vi "Create StringMsg.vi"(8 "error in (no error)":errorcluster, 10 "Message Data":string, 11 "Message Name":string) -> (0 "error out":errorcluster, 3 "StringMsg out":refnum<class "StringMsg.lvclass">)   [LabVIEW 2018, in "LapDog.Messaging.v3.NativeTypes.lvlib" / "StringMsg.lvclass"]
doc: "Returns a StringMsg object with the given name."
uses:
  StringMsg.lvclass
  T:/git/LapDog.Messaging/src/LapDog.Messaging/Message/Message.lvclass
  StringMsg.lvclass/StringMsg.ctl
  LapDog.Messaging/Message/Message.lvclass
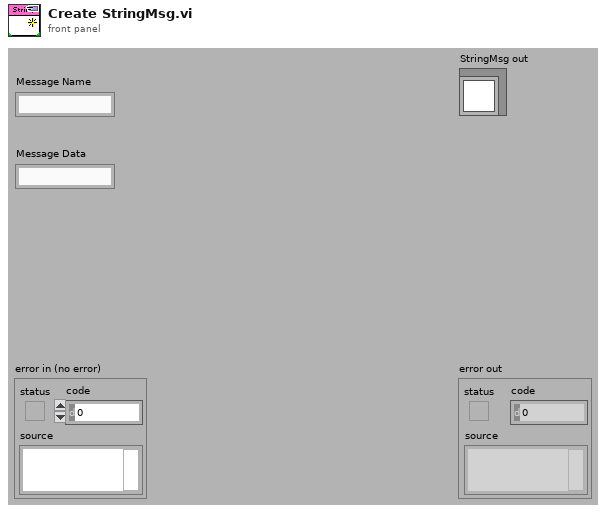
[diagram p1: front panel]
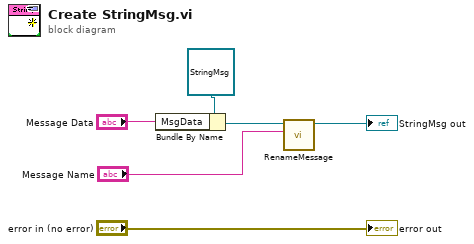
[diagram p0: block diagram]
diagram:
  n1 = Bundle By Name(cluster=refnum<class "StringMsg.lvclass"> refnum ("StringMsg in"), "MsgData"="Message Data") -> (w4:refnum<class "StringMsg.lvclass">)
  n2 = call "RenameMessage.vi"("Message Name"="Message Name", "Message in"=w4) -> ("Message out"=→"StringMsg out":refnum<class "StringMsg.lvclass">)  [unwired: 8 in, 1 out]
  "error out" <- "error in (no error)"
